vi "AlGaAs_SL_v06.vi"(2 "Debug Mode":bool, 3 "Elapsed Time(s)":dbl, 4 "State":enum16{"Edit", "Start", "Run", "End", "Idle"}(ring), 5 "Argument List In":string[](array[string])) -> (0 "Status Out":string, 1 "Argument List Out":string[](array[string]))   [LabVIEW 2011]
panel:
  out "tTotal(s) 2":dbl
  out "is_OK":bool
  out "tTotal(s)":dbl
  out "Do wait 2":bool
  out "Do wait 1":bool
  in  "Tab Control":enum32{"Step 1", "Step 2"}(tab)
  in  "run Ga":bool
  in  "run Al":bool=TRUE
  in  "Al flow":dbl caption="Al flow(0-100sccm)" format="%.1f"
  in  "tFlow(s)":dbl
  in  "tWait(s)":dbl
  in  "Ga flow(0-10sccm)":dbl format="%.3f"
  in  "fGa dilution(>=1)":dbl
  in  "run Ga":bool=TRUE
  in  "run Al":bool
  in  "fGa dilution(>=1)":dbl
  in  "Al flow (0-100sccm)":dbl format="%.1f"
  in  "Ga flow (0-10sccm)":dbl format="%.3f"
  in  "tFlow(s)":dbl
  in  "tWait(s)":dbl
  out "tphase(s)":dbl[](array[numeric])
  out "nstep":dbl
  out "phase":i32
  out "is_done":bool
  in  "nPeriods":dbl
  out "tPeriod(s)":dbl
  in  "Cancel":bool
  in  "OK":bool
  # "Set event time to match total time."
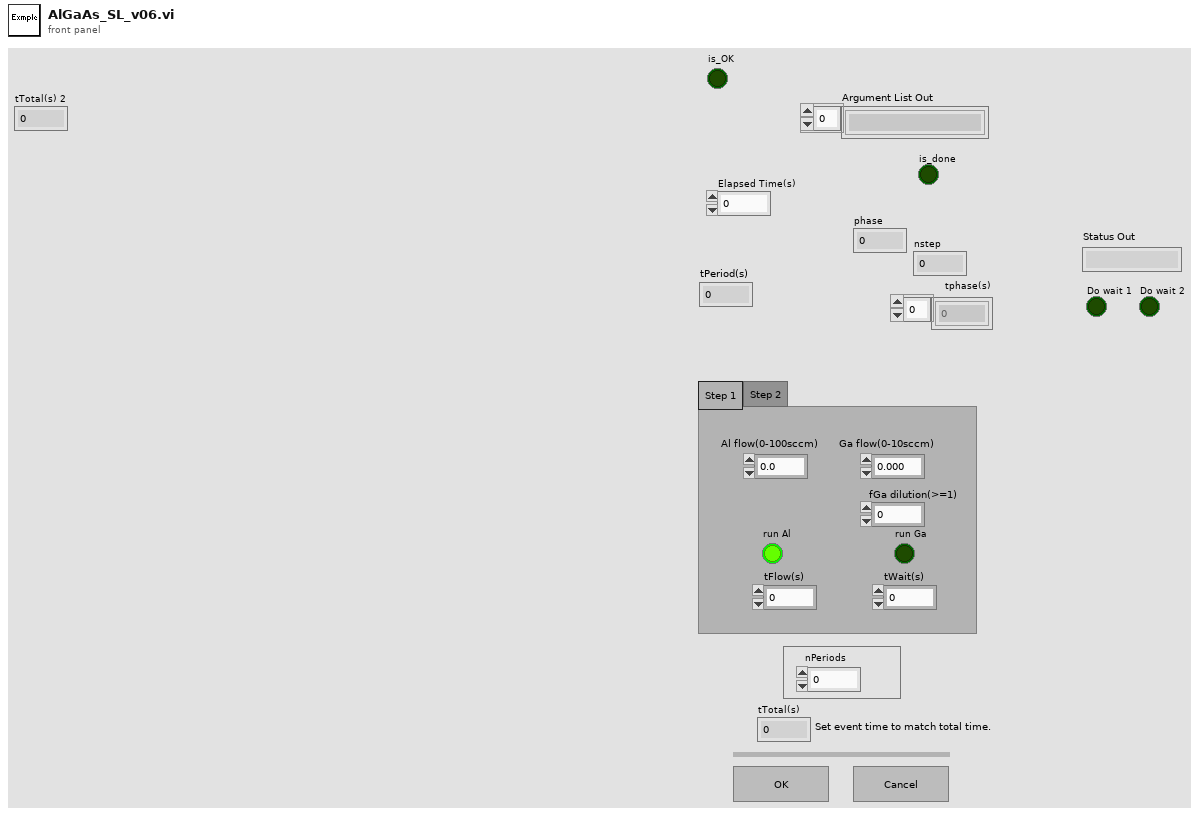
[diagram p1: front panel]
types:
  T1 = enum32{"Invalid", "Default", "Floating", "Floating/Auto-Hide", "Modal"}
  T2 = enum16{"Discrete", "Continuous", "Instantaneous"}
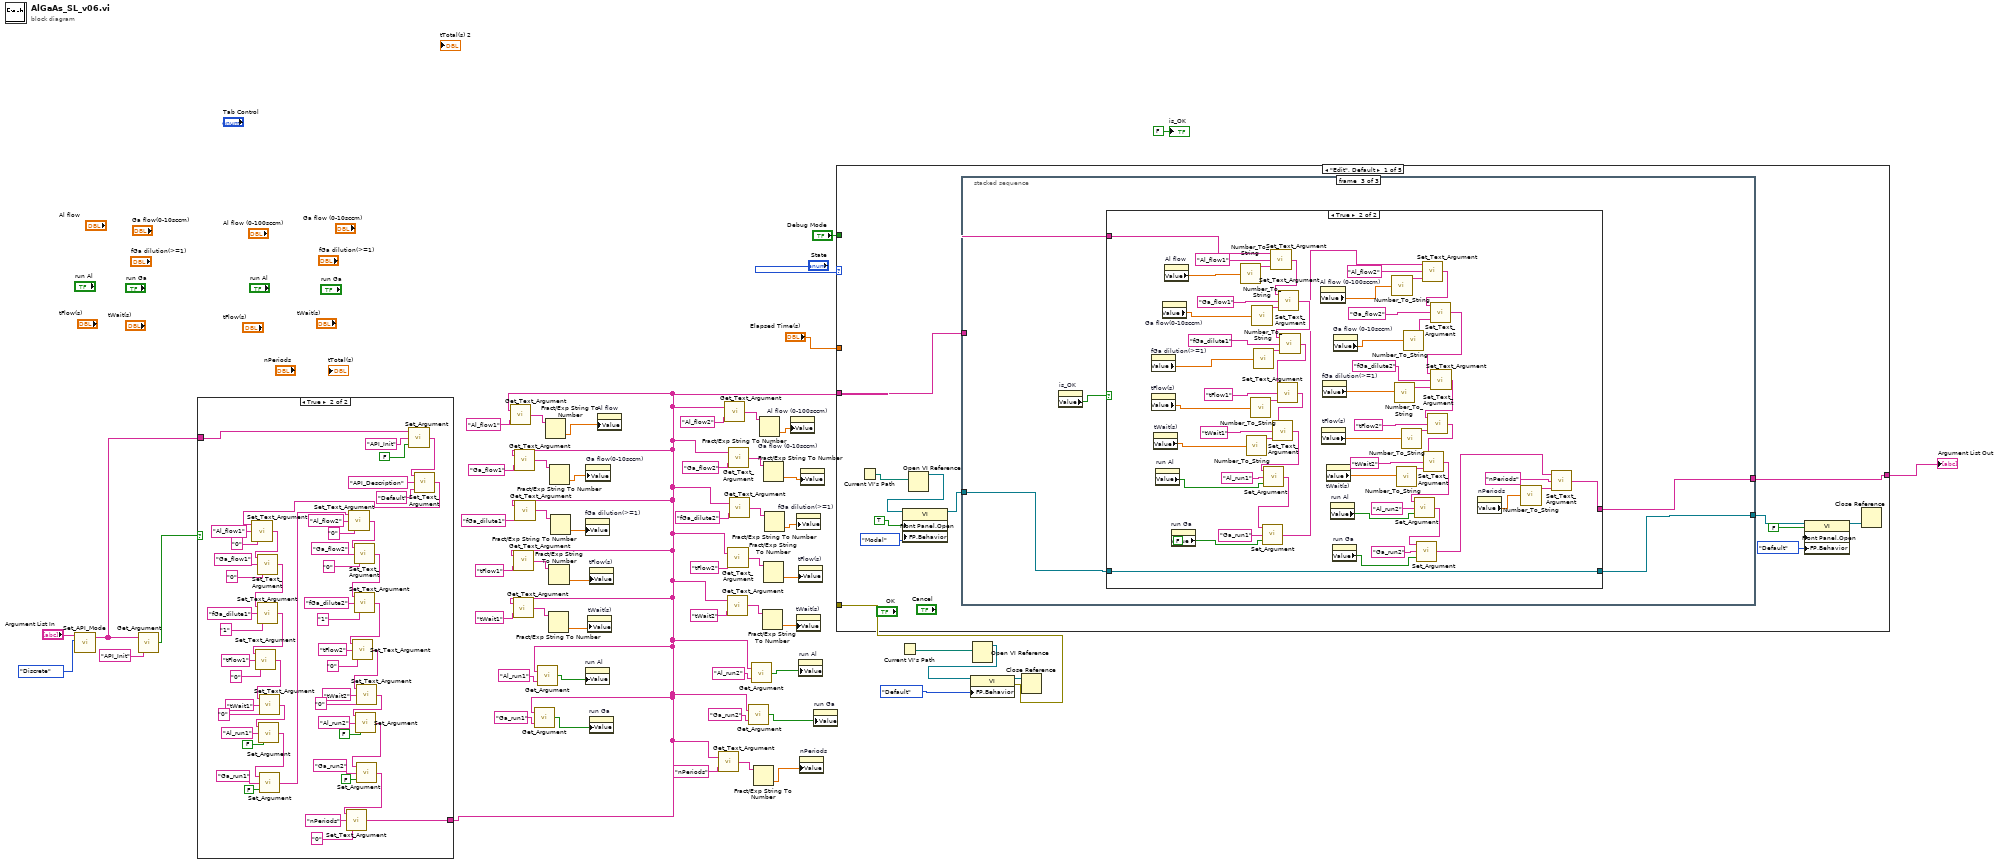
[diagram p0: block diagram]
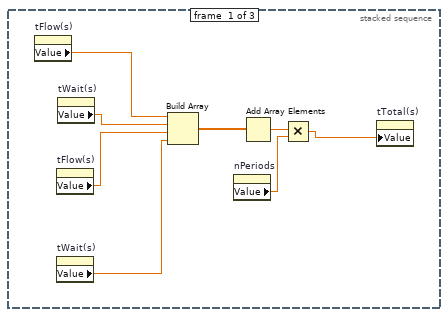
[diagram p3: hidden frame]
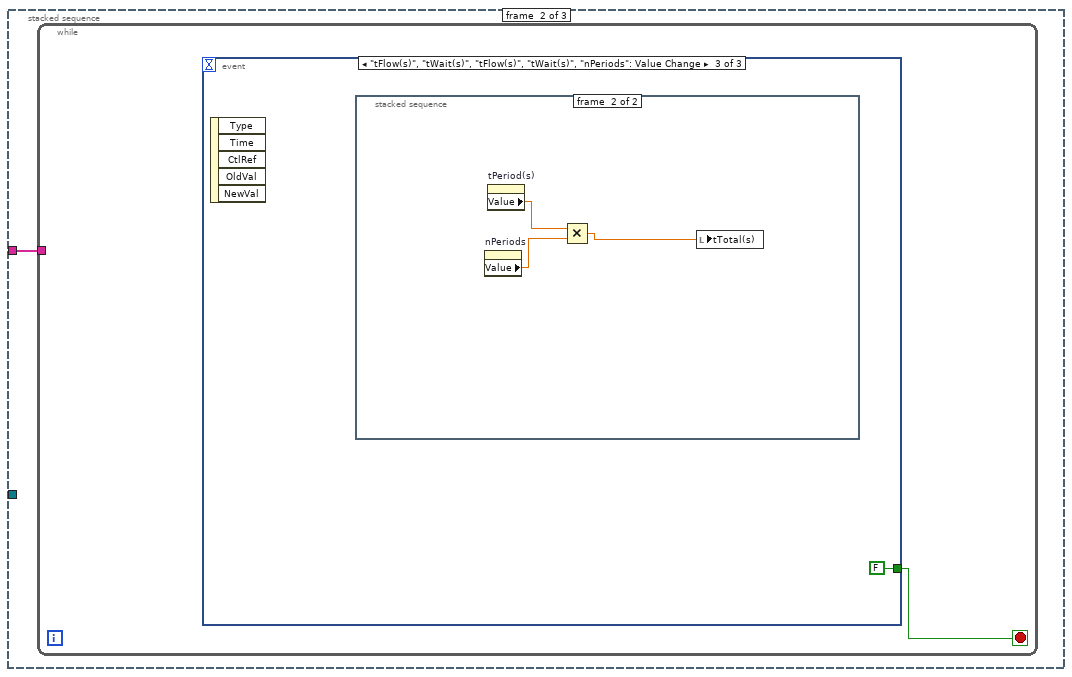
[diagram p4: hidden frame]
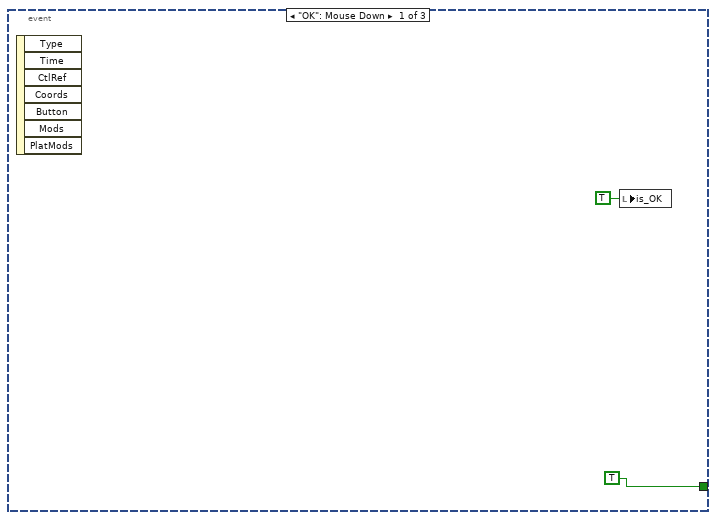
[diagram p5: hidden frame]
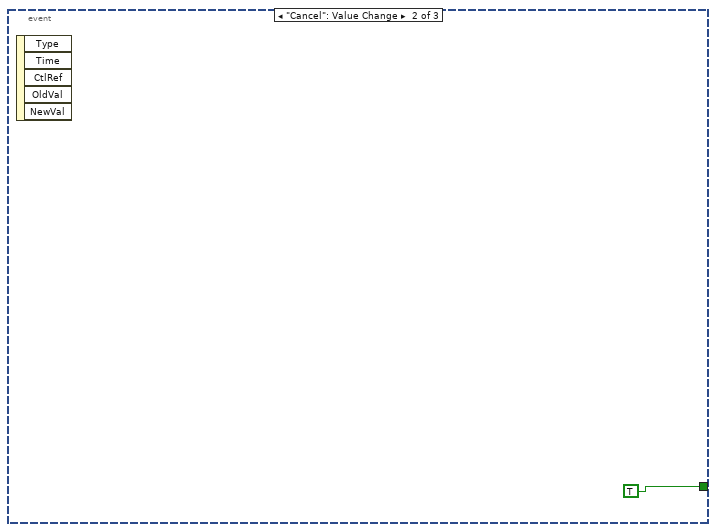
[diagram p6: hidden frame]
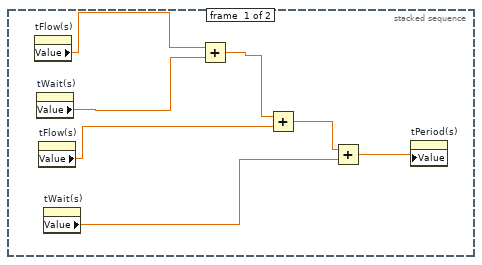
[diagram p7: hidden frame]
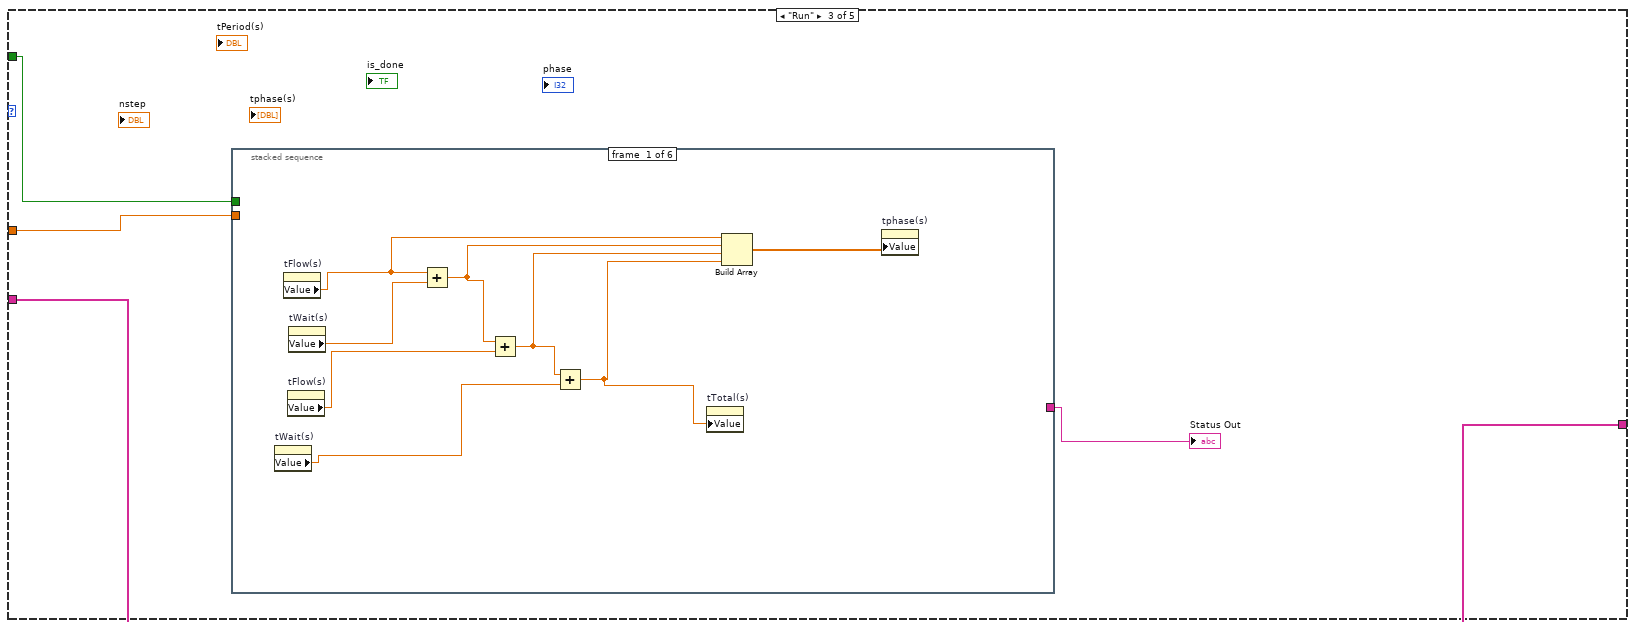
[diagram p10: hidden frame]
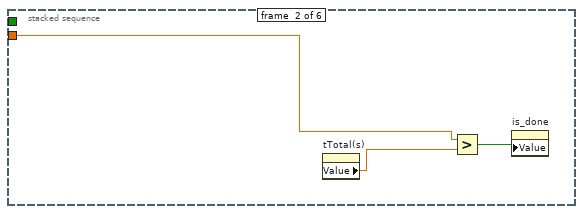
[diagram p11: hidden frame]
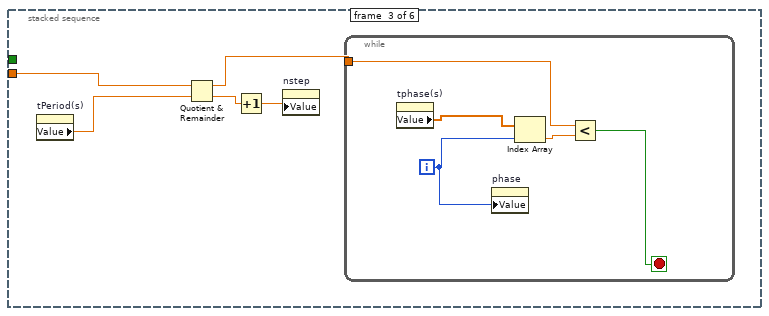
[diagram p12: hidden frame]
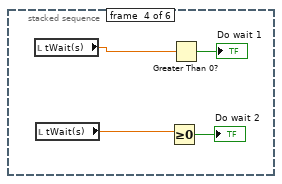
[diagram p13: hidden frame]
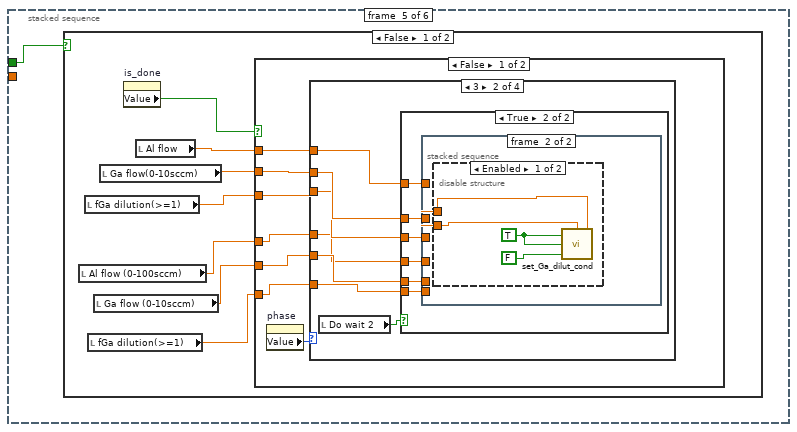
[diagram p14: hidden frame]
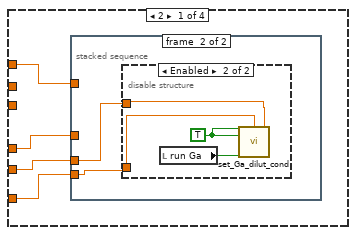
[diagram p15: hidden frame]
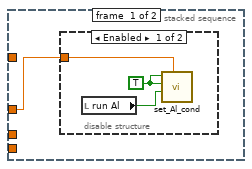
[diagram p16: hidden frame]
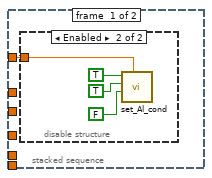
[diagram p20: hidden frame]
diagram:
  n1 = call "Set_API_Mode.vi"("API Mode"=T2."Discrete", "Argument List In"="Argument List In") -> ("Argument List Out"=w51:string[])  [unwired: 3 in]
  n2 = call "Get_Argument.vi"("Argument"="API_Init", "Argument List"=w51) -> ("Enabled"=w50:bool)
  n3 = case shown="True" w50 {
    tunnel: w51 -> [w58 w105]
    tunnel: [w58 w59] -> w8
    frame False {
    }
    frame True {
      n4 = call "Set_Argument.vi"("Enable"=FALSE, "Argument"="API_Init", "Argument List In"=w105) -> ("Argument List Out"=w108:string[])
      n5 = call "Set_Text_Argument.vi"("Text"="Default", "Argument"="API_Description", "Argument List In"=w108) -> ("Argument List Out"=w104:string[])
      n6 = call "Set_Text_Argument.vi"("Text"="0", "Argument"="Al_flow1", "Argument List In"=w104) -> ("Argument List Out"=w89:string[])
      n7 = call "Set_Text_Argument.vi"("Text"="0", "Argument"="Ga_flow1", "Argument List In"=w89) -> ("Argument List Out"=w88:string[])
      n8 = call "Set_Text_Argument.vi"("Text"="1", "Argument"="fGa_dilute1", "Argument List In"=w88) -> ("Argument List Out"=w87:string[])
      n9 = call "Set_Text_Argument.vi"("Text"="0", "Argument"="tFlow1", "Argument List In"=w87) -> ("Argument List Out"=w86:string[])
      n10 = call "Set_Text_Argument.vi"("Text"="0", "Argument"="tWait1", "Argument List In"=w86) -> ("Argument List Out"=w85:string[])
      n11 = call "Set_Argument.vi"("Enable"=FALSE, "Argument"="Al_run1", "Argument List In"=w85) -> ("Argument List Out"=w84:string[])
      n12 = call "Set_Argument.vi"("Enable"=FALSE, "Argument"="Ga_run1", "Argument List In"=w84) -> ("Argument List Out"=w63:string[])
      n13 = call "Set_Text_Argument.vi"("Text"="0", "Argument"="Al_flow2", "Argument List In"=w63) -> ("Argument List Out"=w69:string[])
      n14 = call "Set_Text_Argument.vi"("Text"="0", "Argument"="Ga_flow2", "Argument List In"=w69) -> ("Argument List Out"=w68:string[])
      n15 = call "Set_Text_Argument.vi"("Text"="1", "Argument"="fGa_dilute2", "Argument List In"=w68) -> ("Argument List Out"=w67:string[])
      n16 = call "Set_Text_Argument.vi"("Text"="0", "Argument"="tFlow2", "Argument List In"=w67) -> ("Argument List Out"=w66:string[])
      n17 = call "Set_Text_Argument.vi"("Text"="0", "Argument"="tWait2", "Argument List In"=w66) -> ("Argument List Out"=w65:string[])
      n18 = call "Set_Argument.vi"("Enable"=FALSE, "Argument"="Al_run2", "Argument List In"=w65) -> ("Argument List Out"=w64:string[])
      n19 = call "Set_Argument.vi"("Enable"=FALSE, "Argument"="Ga_run2", "Argument List In"=w64) -> ("Argument List Out"=w60:string[])
      n20 = call "Set_Text_Argument.vi"("Text"="0", "Argument"="nPeriods", "Argument List In"=w60) -> ("Argument List Out"=w59:string[])
    }
  }
  n21 = call "Get_Text_Argument.vi"("Argument"="Al_flow1", "Argument List"=w8) -> ("Text"=w48:string)
  n22 = call "Get_Text_Argument.vi"("Argument"="tWait1", "Argument List"=w8) -> ("Text"=w41:string)
  n23 = call "Get_Text_Argument.vi"("Argument"="tFlow1", "Argument List"=w8) -> ("Text"=w42:string)
  n24 = call "Get_Text_Argument.vi"("Argument"="Ga_flow1", "Argument List"=w8) -> ("Text"=w46:string)
  n25 = call "Get_Text_Argument.vi"("Argument"="fGa_dilute1", "Argument List"=w8) -> ("Text"=w44:string)
  n26 = call "Get_Argument.vi"("Argument"="Ga_run1", "Argument List"=w8) -> ("Enabled"=w17:bool)
  n27 = call "Get_Argument.vi"("Argument"="Al_run1", "Argument List"=w8) -> ("Enabled"=w18:bool)
  n28 = Fract/Exp String To Number(string=w48) -> (number=w23:dbl)  [unwired: 4 out]
  n29 = Fract/Exp String To Number(string=w41) -> (number=w19:dbl)  [unwired: 4 out]
  n30 = Fract/Exp String To Number(string=w42) -> (number=w20:dbl)  [unwired: 4 out]
  n31 = Fract/Exp String To Number(string=w46) -> (number=w22:dbl)  [unwired: 4 out]
  n32 = Fract/Exp String To Number(string=w44) -> (number=w21:dbl)  [unwired: 4 out]
  n33 = property on="fGa dilution(>=1)" class="DigNum (strict)"("Value"=w21) -> ()  [unwired: 2 in, 2 out]
  n34 = property on="run Al" class="Bool (strict)"("Value"=w18) -> ()  [unwired: 2 in, 2 out]
  n35 = property on="Ga flow(0-10sccm)" class="DigNum (strict)"("Value"=w22) -> ()  [unwired: 2 in, 2 out]
  n36 = property on="tWait(s)" class="DigNum (strict)"("Value"=w19) -> ()  [unwired: 2 in, 2 out]
  n37 = property on="tFlow(s)" class="DigNum (strict)"("Value"=w20) -> ()  [unwired: 2 in, 2 out]
  n38 = property on="run Ga" class="Bool (strict)"("Value"=w17) -> ()  [unwired: 2 in, 2 out]
  n39 = property on="Al flow" class="DigNum (strict)"("Value"=w23) -> ()  [unwired: 2 in, 2 out]
  n40 = call "Get_Text_Argument.vi"("Argument"="nPeriods", "Argument List"=w8) -> ("Text"=w25:string)
  n41 = call "Get_Text_Argument.vi"("Argument"="Al_flow2", "Argument List"=w8) -> ("Text"=w36:string)
  n42 = call "Get_Text_Argument.vi"("Argument"="tWait2", "Argument List"=w8) -> ("Text"=w29:string)
  n43 = call "Get_Text_Argument.vi"("Argument"="tFlow2", "Argument List"=w8) -> ("Text"=w30:string)
  n44 = call "Get_Text_Argument.vi"("Argument"="Ga_flow2", "Argument List"=w8) -> ("Text"=w34:string)
  n45 = call "Get_Text_Argument.vi"("Argument"="fGa_dilute2", "Argument List"=w8) -> ("Text"=w32:string)
  n46 = call "Get_Argument.vi"("Argument"="Ga_run2", "Argument List"=w8) -> ("Enabled"=w10:bool)
  n47 = call "Get_Argument.vi"("Argument"="Al_run2", "Argument List"=w8) -> ("Enabled"=w11:bool)
  n48 = Fract/Exp String To Number(string=w25) -> (number=w9:dbl)  [unwired: 4 out]
  n49 = Fract/Exp String To Number(string=w36) -> (number=w16:dbl)  [unwired: 4 out]
  n50 = Fract/Exp String To Number(string=w29) -> (number=w12:dbl)  [unwired: 4 out]
  n51 = Fract/Exp String To Number(string=w30) -> (number=w13:dbl)  [unwired: 4 out]
  n52 = Fract/Exp String To Number(string=w34) -> (number=w15:dbl)  [unwired: 4 out]
  n53 = Fract/Exp String To Number(string=w32) -> (number=w14:dbl)  [unwired: 4 out]
  n54 = property on="Al flow (0-100sccm)" class="DigNum (strict)"("Value"=w16) -> ()  [unwired: 2 in, 2 out]
  n55 = property on="tWait(s)" class="DigNum (strict)"("Value"=w12) -> ()  [unwired: 2 in, 2 out]
  n56 = property on="fGa dilution(>=1)" class="DigNum (strict)"("Value"=w14) -> ()  [unwired: 2 in, 2 out]
  n57 = property on="tFlow(s)" class="DigNum (strict)"("Value"=w13) -> ()  [unwired: 2 in, 2 out]
  n58 = property on="run Al" class="Bool (strict)"("Value"=w11) -> ()  [unwired: 2 in, 2 out]
  n59 = property on="nPeriods" class="DigNum (strict)"("Value"=w9) -> ()  [unwired: 2 in, 2 out]
  n60 = property on="Ga flow (0-10sccm)" class="DigNum (strict)"("Value"=w15) -> ()  [unwired: 2 in, 2 out]
  n61 = property on="run Ga" class="Bool (strict)"("Value"=w10) -> ()  [unwired: 2 in, 2 out]
  n62 = Current VI's Path() -> (path=w6:path)
  n63 = Open VI Reference(vi path=w6) -> (vi reference=w5:refnum<vi>)  [unwired: 1 in, 5 out]
  n64 = property class="VI"(reference=w5, "FP.Behavior"=T1."Default" ("Front Panel Window:Behavior")) -> (reference out=w3:refnum<vi>, error out=w2:errorcluster)  [unwired: 1 in]
  n65 = case shown="\"Edit\", Default" "State" {
    tunnel: "Debug Mode" -> [_ _ w214 _ _]
    tunnel: "Elapsed Time(s)" -> [_ _ w215 _ _]
    tunnel: w8 -> [w121 w211 w212 w388 w389]
    tunnel: [w117 w211 w212 w388 w389] -> w7
    tunnel: w2 -> [_ _ _ _ _]
    frame "Edit", Default {
      n66 = Current VI's Path() -> (path=w115:path)
      n67 = Open VI Reference(vi path=w115) -> (vi reference=w114:refnum<vi>)  [unwired: 1 in, 5 out]
      n68 = property class="VI"(reference=w114, "Front Panel.Open"=TRUE ("Front Panel Window:Open"), "FP.Behavior"=T1."Modal" ("Front Panel Window:Behavior")) -> (reference out=w113:refnum<vi>)  [unwired: 1 in, 1 out]
      n69 = stacked-sequence {
        tunnel: w121 -> [_ w130 w150]
        tunnel: w113 -> [_ _ w147]
        tunnel: [_ _ w146] -> w118
        tunnel: [_ _ w149] -> w117
        frame #0 {
          n70 = property on="tFlow(s)" class="DigNum (strict)"() -> ("Value"=w122:dbl)  [unwired: 2 in, 2 out]
          n71 = property on="tFlow(s)" class="DigNum (strict)"() -> ("Value"=w124:dbl)  [unwired: 2 in, 2 out]
          n72 = property on="tWait(s)" class="DigNum (strict)"() -> ("Value"=w125:dbl)  [unwired: 2 in, 2 out]
          n73 = property on="tWait(s)" class="DigNum (strict)"() -> ("Value"=w123:dbl)  [unwired: 2 in, 2 out]
          n74 = Build Array(w122, w123, w124, w125) -> (w126:dbl[])
          n75 = property on="nPeriods" class="DigNum (strict)"() -> ("Value"=w128:dbl)  [unwired: 2 in, 2 out]
          n76 = Add Array Elements(numeric array=w126) -> (sum=w127:dbl)
          n77 = Multiply(x=w127, y=w128) -> (x*y=w129:dbl)
          n78 = property on="tTotal(s)" class="DigNum (strict)"("Value"=w129) -> ()  [unwired: 2 in, 2 out]
        }
        frame #1 {
          n79 = while {
            tunnel: w130 -> [_]
            stop <- w131 stop-if-true
            n80 = event shown="[2] \"tFlow(s)\", \"tWait(s)\", \"tFlow(s)\", \"tWait(s)\", \"nPeriods\": Value Change" {
              selector: _ -> [_ _ _]
              dyn-events: _ -> [_ _ _]
              timeout: _ -> [_ _ _]
              tunnel: [TRUE ("done_editing") TRUE ("done_editing") FALSE ("done_editing")] -> w131
              event "OK": Mouse Down {
                n81 = event-data() -> ()  [unwired: 1 in, 7 out]
                n82 = local write "is_OK"(TRUE ("is_OK")) -> ()
              }
              event "Cancel": Value Change {
                n83 = event-data() -> ()  [unwired: 1 in, 5 out]
              }
              event "tFlow(s)", "tWait(s)", "tFlow(s)", "tWait(s)", "nPeriods": Value Change {
                n84 = event-data() -> ()  [unwired: 1 in, 5 out]
                n85 = stacked-sequence {
                  frame #0 {
                    n86 = property on="tFlow(s)" class="DigNum (strict)"() -> ("Value"=w139:dbl)  [unwired: 2 in, 2 out]
                    n87 = property on="tWait(s)" class="DigNum (strict)"() -> ("Value"=w140:dbl)  [unwired: 2 in, 2 out]
                    n88 = property on="tFlow(s)" class="DigNum (strict)"() -> ("Value"=w141:dbl)  [unwired: 2 in, 2 out]
                    n89 = property on="tWait(s)" class="DigNum (strict)"() -> ("Value"=w136:dbl)  [unwired: 2 in, 2 out]
                    n90 = Add(x=w139, y=w140) -> (x+y=w138:dbl)
                    n91 = Add(x=w138, y=w141) -> (x+y=w137:dbl)
                    n92 = Add(x=w137, y=w136) -> (x+y=w142:dbl)
                    n93 = property on="tPeriod(s)" class="DigNum (strict)"("Value"=w142) -> ()  [unwired: 2 in, 2 out]
                  }
                  frame #1 {
                    n94 = property on="nPeriods" class="DigNum (strict)"() -> ("Value"=w144:dbl)  [unwired: 2 in, 2 out]
                    n95 = property on="tPeriod(s)" class="DigNum (strict)"() -> ("Value"=w145:dbl)  [unwired: 2 in, 2 out]
                    n96 = Multiply(x=w145, y=w144) -> (x*y=w143:dbl)
                    n97 = local write "tTotal(s)"(w143) -> ()
                  }
                }
              }
            }
          }
        }
        frame #2 {
          n98 = property on="is_OK" class="Bool (strict)"() -> ("Value"=w148:bool)  [unwired: 2 in, 2 out]
          n99 = case shown="True" w148 {
            tunnel: w150 -> [w152 w156]
            tunnel: [w152 w155] -> w149
            tunnel: w147 -> [w151 w154]
            tunnel: [w151 w154] -> w146
            frame False {
            }
            frame True {
              (unwired) FALSE ("is_OK")
              n100 = property on="fGa dilution(>=1)" class="DigNum (strict)"() -> ("Value"=w190:dbl)  [unwired: 2 in, 2 out]
              n101 = property on="tFlow(s)" class="DigNum (strict)"() -> ("Value"=w189:dbl)  [unwired: 2 in, 2 out]
              n102 = property on="tWait(s)" class="DigNum (strict)"() -> ("Value"=w188:dbl)  [unwired: 2 in, 2 out]
              n103 = property on="run Al" class="Bool (strict)"() -> ("Value"=w187:bool)  [unwired: 2 in, 2 out]
              n104 = property on="Ga flow(0-10sccm)" class="DigNum (strict)"() -> ("Value"=w191:dbl)  [unwired: 2 in, 2 out]
              n105 = property on="Al flow" class="DigNum (strict)"() -> ("Value"=w208:dbl)  [unwired: 2 in, 2 out]
              n106 = property on="run Ga" class="Bool (strict)"() -> ("Value"=w186:bool)  [unwired: 2 in, 2 out]
              n107 = call "Number_To_String.vi"("Number"=w208) -> ("String"=w209:string)
              n108 = call "Number_To_String.vi"("Number"=w188) -> ("String"=w200:string)
              n109 = call "Number_To_String.vi"("Number"=w189) -> ("String"=w202:string)
              n110 = call "Number_To_String.vi"("Number"=w191) -> ("String"=w206:string)
              n111 = call "Number_To_String.vi"("Number"=w190) -> ("String"=w204:string)
              n112 = call "Set_Text_Argument.vi"("Text"=w209, "Argument"="Al_flow1", "Argument List In"=w156) -> ("Argument List Out"=w197:string[])
              n113 = call "Set_Text_Argument.vi"("Text"=w206, "Argument"="Ga_flow1", "Argument List In"=w197) -> ("Argument List Out"=w196:string[])
              n114 = call "Set_Text_Argument.vi"("Text"=w204, "Argument"="fGa_dilute1", "Argument List In"=w196) -> ("Argument List Out"=w195:string[])
              n115 = call "Set_Text_Argument.vi"("Text"=w202, "Argument"="tFlow1", "Argument List In"=w195) -> ("Argument List Out"=w194:string[])
              n116 = call "Set_Text_Argument.vi"("Text"=w200, "Argument"="tWait1", "Argument List In"=w194) -> ("Argument List Out"=w193:string[])
              n117 = call "Set_Argument.vi"("Enable"=w187, "Argument"="Al_run1", "Argument List In"=w193) -> ("Argument List Out"=w192:string[])
              n118 = call "Set_Argument.vi"("Enable"=w186, "Argument"="Ga_run1", "Argument List In"=w192) -> ("Argument List Out"=w167:string[])
              n119 = property on="Al flow (0-100sccm)" class="DigNum (strict)"() -> ("Value"=w166:dbl)  [unwired: 2 in, 2 out]
              n120 = property on="tFlow(s)" class="DigNum (strict)"() -> ("Value"=w163:dbl)  [unwired: 2 in, 2 out]
              n121 = property on="fGa dilution(>=1)" class="DigNum (strict)"() -> ("Value"=w164:dbl)  [unwired: 2 in, 2 out]
              n122 = property on="tWait(s)" class="DigNum (strict)"() -> ("Value"=w162:dbl)  [unwired: 2 in, 2 out]
              n123 = property on="run Al" class="Bool (strict)"() -> ("Value"=w161:bool)  [unwired: 2 in, 2 out]
              n124 = property on="run Ga" class="Bool (strict)"() -> ("Value"=w153:bool)  [unwired: 2 in, 2 out]
              n125 = property on="Ga flow (0-10sccm)" class="DigNum (strict)"() -> ("Value"=w165:dbl)  [unwired: 2 in, 2 out]
              n126 = call "Number_To_String.vi"("Number"=w166) -> ("String"=w184:string)
              n127 = call "Number_To_String.vi"("Number"=w164) -> ("String"=w180:string)
              n128 = call "Number_To_String.vi"("Number"=w162) -> ("String"=w176:string)
              n129 = call "Number_To_String.vi"("Number"=w163) -> ("String"=w178:string)
              n130 = call "Number_To_String.vi"("Number"=w165) -> ("String"=w182:string)
              n131 = call "Set_Text_Argument.vi"("Text"=w184, "Argument"="Al_flow2", "Argument List In"=w167) -> ("Argument List Out"=w173:string[])
              n132 = call "Set_Text_Argument.vi"("Text"=w182, "Argument"="Ga_flow2", "Argument List In"=w173) -> ("Argument List Out"=w172:string[])
              n133 = call "Set_Text_Argument.vi"("Text"=w180, "Argument"="fGa_dilute2", "Argument List In"=w172) -> ("Argument List Out"=w171:string[])
              n134 = call "Set_Text_Argument.vi"("Text"=w178, "Argument"="tFlow2", "Argument List In"=w171) -> ("Argument List Out"=w170:string[])
              n135 = call "Set_Text_Argument.vi"("Text"=w176, "Argument"="tWait2", "Argument List In"=w170) -> ("Argument List Out"=w169:string[])
              n136 = call "Set_Argument.vi"("Enable"=w161, "Argument"="Al_run2", "Argument List In"=w169) -> ("Argument List Out"=w168:string[])
              n137 = call "Set_Argument.vi"("Enable"=w153, "Argument"="Ga_run2", "Argument List In"=w168) -> ("Argument List Out"=w157:string[])
              n138 = property on="nPeriods" class="DigNum (strict)"() -> ("Value"=w159:dbl)  [unwired: 2 in, 2 out]
              n139 = call "Number_To_String.vi"("Number"=w159) -> ("String"=w160:string)
              n140 = call "Set_Text_Argument.vi"("Text"=w160, "Argument"="nPeriods", "Argument List In"=w157) -> ("Argument List Out"=w155:string[])
            }
          }
        }
      }
      n141 = property class="VI"(reference=w118, "Front Panel.Open"=FALSE ("Front Panel Window:Open"), "FP.Behavior"=T1."Default" ("Front Panel Window:Behavior")) -> (reference out=w119:refnum<vi>)  [unwired: 1 in, 1 out]
      n142 = Close Reference(reference=w119) -> ()  [unwired: 1 in, 1 out]
    }
    frame "Start" {
    }
    frame "Run" {
      n143 = stacked-sequence {
        tunnel: w215 -> [_ w224 w231 _ _ _]
        tunnel: w214 -> [_ _ _ _ w241 _]
        tunnel: [_ _ _ _ _ w340] -> w213
        frame #0 {
          n144 = property on="tWait(s)" class="DigNum (strict)"() -> ("Value"=w217:dbl)  [unwired: 2 in, 2 out]
          n145 = property on="tFlow(s)" class="DigNum (strict)"() -> ("Value"=w220:dbl)  [unwired: 2 in, 2 out]
          n146 = property on="tFlow(s)" class="DigNum (strict)"() -> ("Value"=w218:dbl)  [unwired: 2 in, 2 out]
          n147 = property on="tWait(s)" class="DigNum (strict)"() -> ("Value"=w219:dbl)  [unwired: 2 in, 2 out]
          n148 = Add(x=w220, y=w219) -> (x+y=w223:dbl)
          n149 = Add(x=w223, y=w218) -> (x+y=w222:dbl)
          n150 = Add(x=w222, y=w217) -> (x+y=w216:dbl)
          n151 = property on="tTotal(s)" class="DigNum (strict)"("Value"=w216) -> ()  [unwired: 2 in, 2 out]
          n152 = Build Array(w220, w223, w222, w216) -> (w221:dbl[])
          n153 = property on="tphase(s)" class="Arr (strict)"("Value"=w221) -> ()  [unwired: 2 in, 2 out]
        }
        frame #1 {
          n154 = property on="tTotal(s)" class="DigNum (strict)"() -> ("Value"=w225:dbl)  [unwired: 2 in, 2 out]
          n155 = Greater?(x=w224, y=w225) -> (0:w226:bool)
          n156 = property on="is_done" class="Bool (strict)"("Value"=w226) -> ()  [unwired: 2 in, 2 out]
        }
        frame #2 {
          n157 = property on="tPeriod(s)" class="DigNum (strict)"() -> ("Value"=w230:dbl)  [unwired: 2 in, 2 out]
          n158 = Quotient & Remainder(x=w231, y=w230) -> (x-y*floor(x/y)=w229:dbl, floor(x/y)=w228:dbl)
          n159 = Increment(x=w228) -> (x+1=w227:dbl)
          n160 = property on="nstep" class="DigNum (strict)"("Value"=w227) -> ()  [unwired: 2 in, 2 out]
          n161 = while {
            tunnel: w229 -> [w235]
            i -> [w233]
            stop <- w232 stop-if-true
            n162 = property on="tphase(s)" class="Arr (strict)"() -> ("Value"=w236:dbl[])  [unwired: 2 in, 2 out]
            n163 = property on="phase" class="DigNum (strict)"("Value"=w233) -> ()  [unwired: 2 in, 2 out]
            n164 = Index Array(array=w236, index=w233) -> (element=w234:dbl)
            n165 = Less?(x=w235, y=w234) -> (x < y?=w232:bool)
          }
        }
        frame #3 {
          n166 = local read "tWait(s)"() -> (w240:dbl)
          n167 = local read "tWait(s)"() -> (w238:dbl)
          n168 = Greater Or Equal To 0?(x=w238) -> (x >= 0?=→"Do wait 2":bool)
          n169 = Greater Than 0?(x=w240) -> (x > 0?=→"Do wait 1":bool)
        }
        frame #4 {
          n170 = case shown="False" w241 {
            frame False {
              n171 = local read "Al flow (0-100sccm)"() -> (w243:dbl)
              n172 = local read "fGa dilution(>=1)"() -> (w244:dbl)
              n173 = local read "fGa dilution(>=1)"() -> (w242:dbl)
              n174 = local read "Ga flow (0-10sccm)"() -> (w248:dbl)
              n175 = local read "Ga flow(0-10sccm)"() -> (w245:dbl)
              n176 = property on="is_done" class="Bool (strict)"() -> ("Value"=w246:bool)  [unwired: 2 in, 2 out]
              n177 = local read "Al flow"() -> (w247:dbl)
              n178 = case shown="False" w246 {
                tunnel: w248 -> [w255 w330]
                tunnel: w247 -> [w254 w331]
                tunnel: w245 -> [w252 _]
                tunnel: w244 -> [w251 _]
                tunnel: w243 -> [w250 _]
                tunnel: w242 -> [w249 _]
                frame False {
                  n179 = property on="phase" class="DigNum (strict)"() -> ("Value"=w253:i32)  [unwired: 2 in, 2 out]
                  n180 = case shown="3" w253 {
                    tunnel: w254 -> [w259 w276 w296 w313]
                    tunnel: w255 -> [w258 w275 _ w309]
                    tunnel: w252 -> [_ w274 w295 w311]
                    tunnel: w251 -> [_ w273 w294 w312]
                    tunnel: w250 -> [w256 w272 _ w310]
                    tunnel: w249 -> [w257 w271 _ w308]
                    frame 2 {
                      n181 = stacked-sequence {
                        tunnel: w259 -> [_ _]
                        tunnel: w258 -> [_ w265]
                        tunnel: w257 -> [_ w264]
                        tunnel: w256 -> [w260 _]
                        frame #0 {
                          n182 = disable-structure shown="Enabled" {
                            disable-tunnel: w260 -> [w263 _]
                            frame Enabled {
                              w262 = TRUE ("Ga Active")
                              n183 = local read "run Al"() -> (w261:bool)
                              n184 = call "set_Al_cond.vi"("Aluminum Flow"=w263, "Al Run"=w261, "Al Bubbler"=w262, "Al Active"=w262) -> ()  [unwired: 6 in]
                            }
                            frame Disabled {
                            }
                          }
                        }
                        frame #1 {
                          n185 = disable-structure shown="Enabled" {
                            disable-tunnel: w265 -> [_ w269]
                            disable-tunnel: w264 -> [_ w268]
                            frame Disabled {
                            }
                            frame Enabled {
                              w267 = TRUE ("Ga Active")
                              n186 = local read "run Ga"() -> (w266:bool)
                              n187 = call "set_Ga_dilut_cond.vi"("Ga flow (0-10 sccm)"=w269, "fDilution"=w268, "Run"=w266, "Bubbler In"=w267, "Active"=w267) -> ()
                            }
                          }
                        }
                      }
                    }
                    frame 3 {
                      n188 = local read "Do wait 2"() -> (w270:bool)
                      n189 = case shown="True" w270 {
                        tunnel: w276 -> [_ w282]
                        tunnel: w275 -> [_ w281]
                        tunnel: w274 -> [_ w280]
                        tunnel: w273 -> [_ w279]
                        tunnel: w272 -> [_ w278]
                        tunnel: w271 -> [_ w277]
                        frame False {
                        }
                        frame True {
                          n190 = stacked-sequence {
                            tunnel: w282 -> [w283 _]
                            tunnel: w281 -> [_ _]
                            tunnel: w280 -> [_ w289]
                            tunnel: w279 -> [_ w288]
                            tunnel: w278 -> [_ _]
                            tunnel: w277 -> [_ _]
                            frame #0 {
                              n191 = disable-structure shown="Enabled" {
                                disable-tunnel: w283 -> [_ w284]
                                frame Disabled {
                                }
                                frame Enabled {
                                n192 = call "set_Al_cond.vi"("Aluminum Flow"=w284, "Al Run"=FALSE, "Al Bubbler"=TRUE, "Al Active"=TRUE) -> ()  [unwired: 6 in]
                                }
                              }
                            }
                            frame #1 {
                              n193 = disable-structure shown="Enabled" {
                                disable-tunnel: w289 -> [w293 _]
                                disable-tunnel: w288 -> [w292 _]
                                frame Enabled {
                                w291 = TRUE ("Ga Active")
                                n194 = call "set_Ga_dilut_cond.vi"("Ga flow (0-10 sccm)"=w293, "fDilution"=w292, "Run"=FALSE ("Ga Run"), "Bubbler In"=w291, "Active"=w291) -> ()
                                }
                                frame Disabled {
                                }
                              }
                            }
                          }
                        }
                      }
                    }
                    frame 0, Default {
                      n195 = stacked-sequence {
                        tunnel: w296 -> [w297 _]
                        tunnel: w295 -> [_ w302]
                        tunnel: w294 -> [_ w301]
                        frame #0 {
                          n196 = disable-structure shown="Enabled" {
                            disable-tunnel: w297 -> [_ w300]
                            frame Disabled {
                            }
                            frame Enabled {
                              w299 = TRUE ("Al Active")
                              n197 = local read "run Al"() -> (w298:bool)
                              n198 = call "set_Al_cond.vi"("Aluminum Flow"=w300, "Al Run"=w298, "Al Bubbler"=w299, "Al Active"=w299) -> ()  [unwired: 6 in]
                            }
                          }
                        }
                        frame #1 {
                          n199 = disable-structure shown="Enabled" {
                            disable-tunnel: w302 -> [w306 _]
                            disable-tunnel: w301 -> [w305 _]
                            frame Enabled {
                              w304 = TRUE ("Ga Active")
                              n200 = local read "run Ga"() -> (w303:bool)
                              n201 = call "set_Ga_dilut_cond.vi"("Ga flow (0-10 sccm)"=w306, "fDilution"=w305, "Run"=w303, "Bubbler In"=w304, "Active"=w304) -> ()
                            }
                            frame Disabled {
                            }
                          }
                        }
                      }
                    }
                    frame 1 {
                      n202 = local read "Do wait 1"() -> (w307:bool)
                      n203 = case shown="True" w307 {
                        tunnel: w313 -> [_ w319]
                        tunnel: w312 -> [_ w318]
                        tunnel: w311 -> [_ w317]
                        tunnel: w310 -> [_ w316]
                        tunnel: w309 -> [_ w315]
                        tunnel: w308 -> [_ w314]
                        frame False {
                        }
                        frame True {
                          n204 = stacked-sequence {
                            tunnel: w319 -> [_ _]
                            tunnel: w318 -> [_ _]
                            tunnel: w317 -> [_ _]
                            tunnel: w316 -> [w320 _]
                            tunnel: w315 -> [_ w324]
                            tunnel: w314 -> [_ w325]
                            frame #0 {
                              n205 = disable-structure shown="Enabled" {
                                disable-tunnel: w320 -> [_ w321]
                                frame Disabled {
                                }
                                frame Enabled {
                                w322 = TRUE ("Al Bubbler")
                                n206 = call "set_Al_cond.vi"("Aluminum Flow"=w321, "Al Run"=FALSE, "Al Bubbler"=w322, "Al Active"=w322) -> ()  [unwired: 6 in]
                                }
                              }
                            }
                            frame #1 {
                              n207 = disable-structure shown="Enabled" {
                                disable-tunnel: w324 -> [w327 _]
                                disable-tunnel: w325 -> [w326 _]
                                frame Enabled {
                                w328 = TRUE ("Ga Active")
                                n208 = call "set_Ga_dilut_cond.vi"("Ga flow (0-10 sccm)"=w327, "fDilution"=w326, "Run"=FALSE ("Ga Run"), "Bubbler In"=w328, "Active"=w328) -> ()
                                }
                                frame Disabled {
                                }
                              }
                            }
                          }
                        }
                      }
                    }
                  }
                }
                frame True {
                  n209 = stacked-sequence {
                    tunnel: w331 -> [w332 _]
                    tunnel: w330 -> [_ w336]
                    frame #0 {
                      n210 = disable-structure shown="Enabled" {
                        disable-tunnel: w332 -> [_ w335]
                        frame Disabled {
                        }
                        frame Enabled {
                          w334 = TRUE ("Al Active")
                          n211 = call "set_Al.vi"("Aluminum Flow"=w335, "Al Run"=FALSE, "Al Bubbler"=w334, "Al Active"=w334) -> ()  [unwired: 6 in]
                        }
                      }
                    }
                    frame #1 {
                      n212 = disable-structure shown="Enabled" {
                        disable-tunnel: w336 -> [w337 _]
                        frame Enabled {
                          w338 = TRUE ("Ga Active")
                          n213 = call "set_Ga.vi"("Ga Active"=w338, "Ga Flow 1"=w337, "Ga Bubbler"=w338, "Ga Run"=FALSE) -> ()  [unwired: 4 in, 8 out]
                        }
                        frame Disabled {
                        }
                      }
                    }
                  }
                }
              }
            }
            frame True {
            }
          }
        }
        frame #5 {
          n214 = property on="is_done" class="Bool (strict)"() -> ("Value"=w341:bool)  [unwired: 2 in, 2 out]
          n215 = case shown="False" w341 {
            tunnel: [w350 w387] -> w340
            frame False {
              w344 = ", " ("string")
              n216 = property on="phase" class="DigNum (strict)"() -> ("Value"=w343:i32)  [unwired: 2 in, 2 out]
              n217 = Increment(x=w343) -> (x+1=w342:i32)
              n218 = Format Into String(format string="%2.0f", w342) -> (resulting string=w348:string)  [unwired: 2 in, 1 out]
              n219 = case shown="3" w343 {
                tunnel: [w358 "wait (after 2)" w369 "wait (after 1)"] -> w345
                frame 2 {
                  n220 = local read "Ga flow (0-10sccm)"() -> (w360:dbl)
                  n221 = local read "Al flow (0-100sccm)"() -> (w361:dbl)
                  n222 = Format Into String(format string="%4.1f", w361) -> (resulting string=w364:string)  [unwired: 2 in, 1 out]
                  n223 = Format Into String(format string="%4.1f", w360) -> (resulting string=w367:string)  [unwired: 2 in, 1 out]
                  n224 = Concatenate Strings("Al(" ("string"), w364, "sccm)" ("string")) -> (w359:string)
                  n225 = Concatenate Strings(w359, "Ga(" ("string"), w367, "sccm)" ("string")) -> (w358:string)
                }
                frame 3 {
                }
                frame 0, Default {
                  n226 = local read "Ga flow(0-10sccm)"() -> (w375:dbl)
                  n227 = local read "Al flow"() -> (w376:dbl)
                  n228 = Format Into String(format string="%4.1f", w376) -> (resulting string=w378:string)  [unwired: 2 in, 1 out]
                  n229 = Format Into String(format string="%4.1f", w375) -> (resulting string=w371:string)  [unwired: 2 in, 1 out]
                  n230 = Concatenate Strings("Al(" ("string"), w378, "sccm)" ("string")) -> (w370:string)
                  n231 = Concatenate Strings(w370, "Ga(" ("string"), w371, "sccm)" ("string")) -> (w369:string)
                }
                frame 1 {
                }
              }
              n232 = Concatenate Strings("Phase " ("string"), w348) -> (w346:string)
              n233 = property on="nstep" class="DigNum (strict)"() -> ("Value"=w355:dbl)  [unwired: 2 in, 2 out]
              n234 = Format Into String(format string="%3.0f", w355) -> (resulting string=w352:string)  [unwired: 2 in, 1 out]
              n235 = Concatenate Strings("Period " ("string"), w352) -> (w351:string)
              n236 = Concatenate Strings(w351, w344, w346, w344, w345) -> (w350:string)
            }
            frame True {
              n237 = property on="nPeriods" class="DigNum (strict)"() -> ("Value"=w382:dbl)  [unwired: 2 in, 2 out]
              n238 = Format Into String(format string="%3.0f", w382) -> (resulting string=w383:string)  [unwired: 2 in, 1 out]
              n239 = Concatenate Strings("done after", w383, " periods" ("string")) -> (w387:string)
            }
          }
        }
      }
      "Status Out" <- w213
    }
    frame "End" {
    }
    frame "Idle" {
    }
  }
  "Argument List Out" <- w7
  n240 = Close Reference(reference=w3) -> ()  [unwired: 1 in, 1 out]
  "is_OK" <- FALSE ("is_OK")
